vi "Pixel Histogram.vi"(11 "input":u16[][][](array[numeric])) -> (1 "Image Size Changed?":bool, 2 "X Values":dbl[](array[numeric]), 3 "Histogram: h(x)":i32[](array[numeric]))   [LabVIEW 2023, in "Viewer.lvlib" / "Viewer.lvclass"]
uses:
  Viewer.lvclass
  Viewer.lvclass/Viewer.ctl
  <vilib>/Analysis/NI_AALBase.lvlib
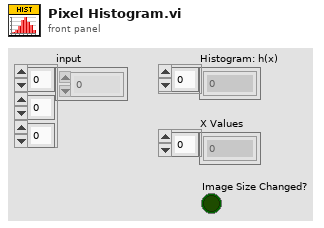
[diagram p1: front panel]
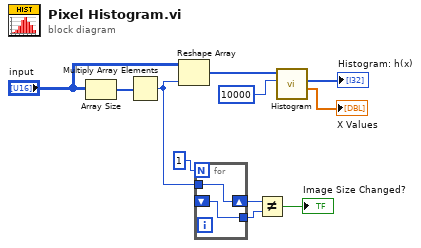
[diagram p0: block diagram]
diagram:
  n1 = Array Size(array="input") -> (size(s)=w8:i32[])
  n2 = Multiply Array Elements(1:w8) -> (0:w5:i32)
  n3 = Reshape Array("input", w5) -> (w7:u16[])
  n4 = for {
    N: 1 -> [_]
    tunnel: w5 -> [w13]
    shift-right: [w13] -> w3
    shift-left: _ -> [w12]
    tunnel: [w12] -> w2
  }
  n5 = Not Equal?(x=w3, y=w2) -> (x != y?=→"Image Size Changed?":bool)
  n6 = call <vilib>:"Histogram.vi"("intervals"=10000, "X"=w7) -> ("X Values"=→"X Values":dbl[], "Histogram: h(x)"=→"Histogram: h(x)":i32[])  [unwired: 6 in, 2 out]
